vi "Transform.vi"(8 "error in (no error)":errorcluster, 11 "XRay Part Sample in":refnum<class "XRay Part Sample.lvclass">=refnum) -> (0 "error out":errorcluster, 3 "XRay Part Sample out":refnum<class "XRay Part Sample.lvclass">)   [LabVIEW 2026, in "XRay Part Sample.lvclass"]
uses:
  XRay Part Sample.lvclass
  XRay Table/XRay Table.lvclass
  XRay Part Sample.lvclass/XRay Part Sample.ctl
  XRay Table/XRay Table.lvclass/XRay Table.ctl
  <vilib>/picture/3D Picture Control/NI_3D Picture Control.lvlib
panel:
  in  "Translation 4":cluster{"X":sgl, "Y":sgl, "Z":sgl}={"X"=1.0, "Y"=-7.0, "Z"=0.0}
  in  "Translation 3":cluster{"X":sgl, "Y":sgl, "Z":sgl}={"X"=0.0, "Y"=3.0, "Z"=0.5}
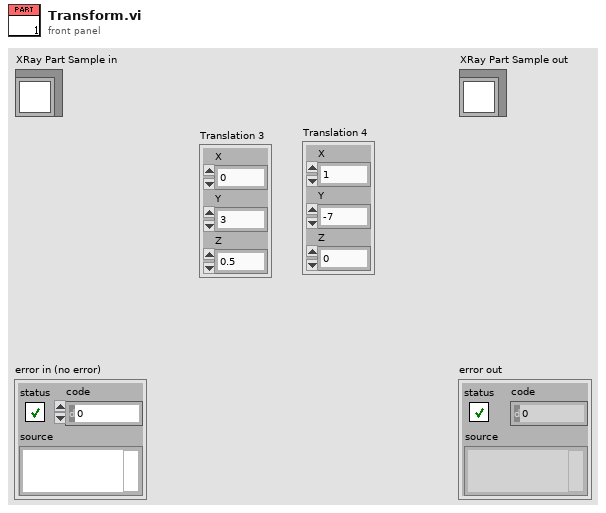
[diagram p1: front panel]
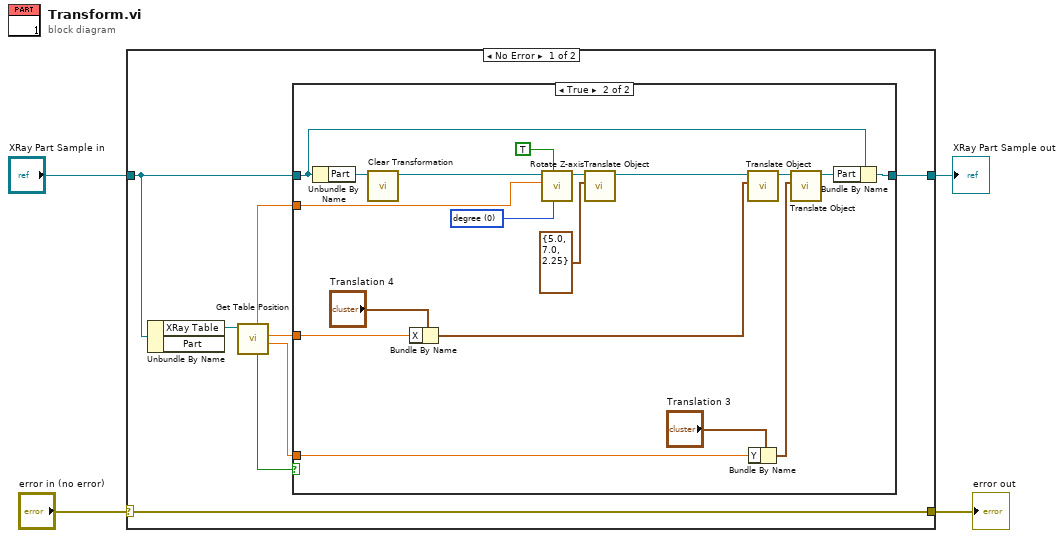
[diagram p0: block diagram]
diagram:
  n1 = case shown="No Error" "error in (no error)" {
    selector: "error in (no error)" -> [w12 w33]
    tunnel: [w12 w33] -> w3
    tunnel: [w9 w32] -> w1
    tunnel: "XRay Part Sample in" -> [w10 w32]
    frame No Error {
      n2 = Unbundle By Name(w10) -> ("XRay Table"=w11:refnum<class "XRay Table.lvclass">)  [unwired: 1 out]
      n3 = call "Get Table Position.vi"("XRay Table in"=w11) -> ("Y Position"=w7:dbl, "X Position"=w8:dbl, "Pos Changed"=w6:bool, "Table Rotation"=w5:dbl)  [unwired: 5 in, 2 out]
      n4 = case shown="True" w6 {
        tunnel: w10 -> [w13 w26]
        tunnel: [w13 w25] -> w9
        tunnel: w8 -> [_ w24]
        tunnel: w7 -> [_ w23]
        tunnel: w5 -> [_ w19]
        frame False {
        }
        frame True {
          w20 = u16 0 items=["degree", "radians"] ("angle unit")
          n5 = Unbundle By Name(w26) -> ("Part"=w31:refnum<vi>)
          n6 = call <vilib>:"Clear Transformation.vi"("Object Refnum In"=w31) -> ("Object Refnum Out"=w18:refnum<vi>)  [unwired: 1 in, 9 out]
          n7 = Bundle By Name(cluster="Translation 4", "X"=w24) -> (w28:cluster{"X":sgl, "Y":sgl, "Z":sgl})
          n8 = call <vilib>:"Rotate Z-axis.vi"("angle unit"=w20, "Relative?"=TRUE, "angle"=w19, "Scene Object In"=w18) -> ("Scene Object Out"=w17:refnum<vi>)  [unwired: 6 in, 1 out]
          n9 = call <vilib>:"Translate Object.vi"("Translation"=cluster{"x":sgl, "y (Zoom)":sgl, "z":sgl} {"x"=5.0, "y (Zoom)"=7.0, "z"=2.25} ("output cluster"), "Scene.Object In"=w17) -> ("Scene.Object Out"=w15:refnum<vi>)  [unwired: 8 in, 1 out]
          n10 = call <vilib>:"Translate Object.vi"("Translation"=w28, "Scene.Object In"=w15) -> ("Scene.Object Out"=w22:refnum<vi>)  [unwired: 8 in, 1 out]
          n11 = Bundle By Name(cluster="Translation 3", "Y"=w23) -> (w29:cluster{"X":sgl, "Y":sgl, "Z":sgl})
          n12 = call <vilib>:"Translate Object.vi"("Translation"=w29, "Scene.Object In"=w22) -> ("Scene.Object Out"=w14:refnum<vi>)  [unwired: 8 in, 1 out]
          n13 = Bundle By Name(cluster=w26, "Part"=w14) -> (w25:refnum<class "XRay Part Sample.lvclass">)
        }
      }
    }
    frame Error {
    }
  }
  "error out" <- w3
  "XRay Part Sample out" <- w1
